vi "LockedHeading.vi"(9 "LockHeading":bool, 11 "Heading In":dbl) -> (3 "LockedHeading":dbl)   [LabVIEW 2015]
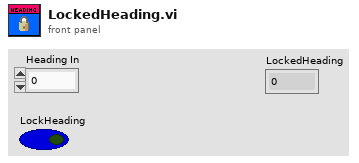
[diagram p1: front panel]
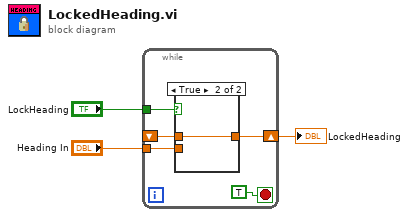
[diagram p0: block diagram]
diagram:
  n1 = while {
    tunnel: "LockHeading" -> [w8]
    tunnel: "Heading In" -> [w6]
    shift-right: [w7] -> w2
    shift-left: _ -> [w5]
    stop <- TRUE stop-if-true
    n2 = case shown="True" w8 {
      tunnel: [w9 w10] -> w7
      tunnel: w6 -> [w9 _]
      tunnel: w5 -> [_ w10]
      frame False {
      }
      frame True {
      }
    }
  }
  "LockedHeading" <- w2
